vi "Read Tag Element (Boolean).vi"(8 "error in":errorcluster, 9 "default":bool, 10 "Tag Name":string, 11 "node in":refnum<k20>) -> (0 "error out":errorcluster, 1 "value":bool, 3 "node out":refnum<k20>)   [LabVIEW 2020, in "ARINC 429 Import.lvlib"]
uses:
  ARINC 429 Import.lvlib
  <resource>/objmgr/DOMUserDefRef.rc
  <vilib>/xml/NI_XML.lvlib
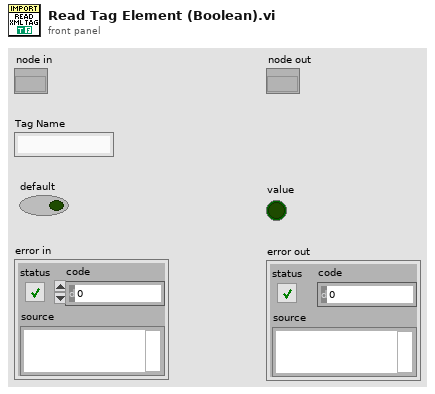
[diagram p1: front panel]
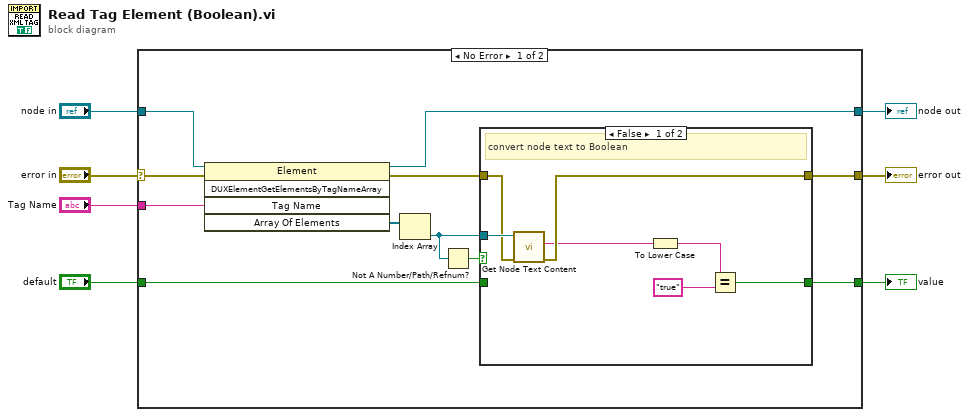
[diagram p0: block diagram]
diagram:
  n1 = case shown="No Error" "error in" {
    selector: "error in" -> [w8 w30]
    tunnel: [w18 w30] -> w7
    tunnel: "node in" -> [w14 w29]
    tunnel: "Tag Name" -> [w12 _]
    tunnel: [w11 w28] -> w4
    tunnel: [w10 w29] -> w3
    tunnel: "default" -> [w9 w28]
    frame No Error {
      n2 = invoke class="Element" method="DUXElementGetElementsByTagNameArray"(reference=w14, error in=w8, "Tag Name"=w12) -> (reference out=w10:refnum<k20>, error out=w17:errorcluster, "Array Of Elements"=w13:refnum<k20>[])  [unwired: 2 in, 2 out]
      n3 = Index Array(array=w13) -> (element=w15:refnum<k20>)  [unwired: 1 in]
      n4 = Not A Number/Path/Refnum?(number/path/refnum=w15) -> (NaN/Path/Refnum?=w16:bool)
      n5 = case shown="False" w16 {
        tunnel: w15 -> [w25 _]
        tunnel: w17 -> [w24 w27]
        tunnel: [w21 w26] -> w11
        tunnel: [w23 w27] -> w18
        tunnel: w9 -> [_ w26]
        frame False {
          # "convert node text to Boolean"
          n6 = call <vilib>:"Get Node Text Content.vi"("error in (no error)"=w24, "node in"=w25) -> ("error out"=w23:errorcluster, "node text"=w22:string)  [unwired: 7 in, 1 out]
          n7 = To Lower Case(string=w22) -> (all lower case string=w19:string)
          n8 = Equal?(x=w19, y="true" ("x")) -> (x = y?=w21:bool)
        }
        frame True {
          # "pass default if element doesn't exist"
        }
      }
    }
    frame Error {
    }
  }
  "error out" <- w7
  "node out" <- w3
  "value" <- w4
